vi "InitDGSystems from CnfgFile HW.vi"(8 "error in":errorcluster, 10 "Dir Calibration files":path, 11 "Config File":path) -> (0 "Errors":errorcluster[](array[cluster]), 1 "new Modules.cal?":bool, 2 "Problem Chnls out":string[](array[string]), 3 "DG Systems":refnum<class "BME_DG_System.lvclass">[](array[class]), 4 "ChnlNames":string[](array[string]), 5 "SystemNames":string[](array[string]))   [LabVIEW 2009, in "POLARIS BME DG.lvlib" / "BME_DG_System.lvclass"]
doc: "VI reads configration file and\n - reserves memory for all installed DGs\n - initializes all found systems\n - calibrates all DGs from Modules.cal\n\nOutput:\n - Problem Chnls Out : contains names of channels, they cause inconsystence by delay formulast\n - DG Systems : Array with initialized BME_DG_Systems object\n - ChnlNames : Array with all channel names in all systems\n - new Modules.cal? : is true if new Modules.cal is created. If it is the case it may by needed to correct values inside this file."
uses:
  BME_DG_System.lvclass
  POLARIS BME DG.lvlib
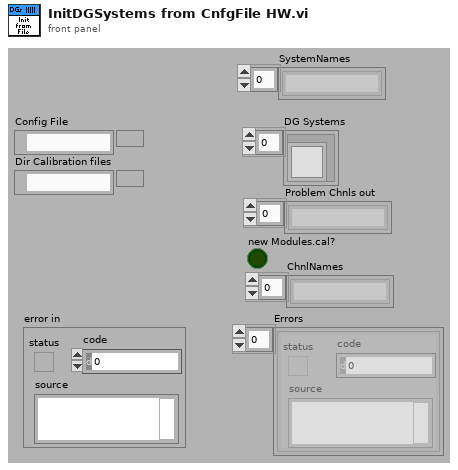
[diagram p1: front panel]
types:
  T1 = typedef "POLARIS BME DG.lvlib/BME_DG_MasterOrSlave.ctl" = enum16{"Unknown", "Master", "Slave"}
  T2 = typedef "POLARIS BME DG.lvlib/System DG Selection.ctl" = cluster{"Selected System DGs":T3[], "Name":string}
  T3 = typedef "POLARIS BME DG.lvlib/DetectDG.ctl" = cluster{"DG_Number":i32, "DG_Product":i32, "Product Name":string, "Bus_Number":i32, "Slot_Number":i32, "Master":bool}
  T4 = typedef "POLARIS BME DG.lvlib/Card Config.ctl" = cluster{"Logical Name":string, "Base Settings":T5, "SG08_Settings":T7, "Channel Names":string[], "Advanced Settings":T8}
  T5 = typedef "POLARIS BME DG.lvlib/BME_DG_TriggerSettings.ctl" = cluster{"Clock Source":T6, " clock modulo":u32, "TriggerEnabled?":bool, "trigger modulo ":i32, "InputTerminated?":bool, "Inhibit(µs)":dbl, "TriggerLevel":dbl, "PresetValue":i32, "InternalTrigger?":bool, "InternalArm?":bool, "SWTrigger?":bool, "RisingEdge?":bool, "StopOnPreset?":bool, "ResetWhenDone?":bool, "Gate Divider":i32, "PositiveGate?":bool}
  T6 = typedef "POLARIS BME DG.lvlib/ClockSource.ctl" = i32
  T7 = typedef "POLARIS BME DG.lvlib/SG08_Settings.ctl" = cluster{"Gate Terminate":bool, "Gate Level":dbl, "Gate Delay (µs)":dbl, "StepBackTime (µs)":dbl, "Burst Counter":u32, "Trigger Divider":u32, "Trigger Multiplier":u32}
  T8 = typedef "POLARIS BME DG.lvlib/BME_DG_V2TriggerSettings.ctl" = cluster{"Trigger on MS Bus":T9, "Force Trigger (µs)":dbl, "Gate Type":bool, "Synchronize Gate":bool}
  T9 = typedef "POLARIS BME DG.lvlib/MSBusSignals.ctl" = u32
  T10 = typedef "POLARIS BME DG.lvlib/Chnl Settings Complete.ctl" = cluster{"Channel Name":string, "ChnParameter":T11, "DelayFormula":string, "OutputModulo":i32, "Go and Done Signal":T12, "G08_Chnl_Settings":T14}
  T11 = typedef "POLARIS BME DG.lvlib/ChnlSettings.ctl" = cluster{" Delay (µs)":dbl, "On?":bool, "PositiveVoltage?":bool, "50OhmTerminated? ":bool, "25OhmOutput?":bool}
  T12 = typedef "POLARIS BME DG.lvlib/Go_Done_Chnl_Settings.ctl" = cluster{"Go Signal":T13, "Done Signal":u32}
  T13 = typedef "POLARIS BME DG.lvlib/GoSignalBits.ctl" = u32
  T14 = typedef "POLARIS BME DG.lvlib/SG08_Chnl_Settings.ctl" = cluster{"Pulse Width (µs)":dbl, "Output Offset":u32, "Disconnect (E,F)":bool, "Onto MsBus (E,F)":bool, "Input Positive (E,F)":bool}
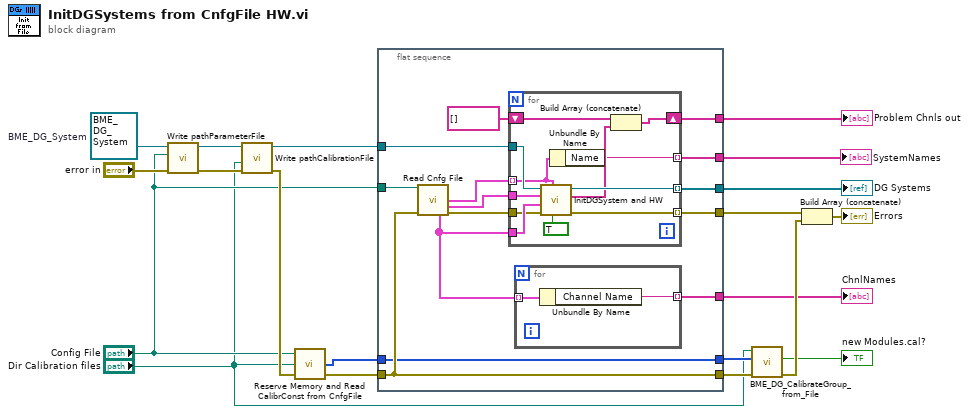
[diagram p0: block diagram]
diagram:
  w18 = refnum<class "BME_DG_System.lvclass"> refnum  # BME_DG_System
  n1 = call-dynamic "Write pathParameterFile.vi"("error in (no error)"="error in", "pathParameterFile"="Config File", "BME_DG_System in"=w18) -> ("error out"=w9:errorcluster, "BME_DG_System out"=w10:refnum<class "BME_DG_System.lvclass">)  [unwired: 7 in]
  n2 = call-dynamic "Write pathCalibrationFile.vi"("error in (no error)"=w9, "pathModulesCal"="Dir Calibration files", "BME_DG_System in"=w10) -> ("error out"=w8:errorcluster, "BME_DG_System out"=w11:refnum<class "BME_DG_System.lvclass">)  [unwired: 7 in]
  n3 = call "Reserve Memory and Read CalibrConst from CnfgFile.vi"("error in"=w8, "pathCalibrConsts"="Dir Calibration files", "pathConfigFile"="Config File") -> ("error out"=w17:errorcluster, "Master or Slave?"=w15:T1[])  [unwired: 1 in]
  n4 = flat-sequence {
    tunnel: [w31] -> w20
    tunnel: [w30] -> w19
    tunnel: w11 -> [w29]
    tunnel: w17 -> [w27]
    tunnel: "Config File" -> [w28]
    tunnel: [w27] -> w16
    tunnel: [w26] -> w14
    tunnel: w15 -> [w26]
    tunnel: [w25] -> w4
    tunnel: [w22] -> w3
    tunnel: [w21] -> w1
    frame #0 {
      n5 = call "Read Cnfg File.vi"("Config File"=w28, "error in (no error)"=w27) -> ("DGSystems"=w34:T2[], "Cards"=w32:T4[], "Chnls"=w23:T10[], "error out"=w33:errorcluster)  [unwired: 8 in, 2 out]
      n6 = for {
        tunnel: w34 -> [w38] mode=indexing
        tunnel: w33 -> [w46]
        tunnel: w32 -> [w48]
        tunnel: w23 -> [w47]
        tunnel: [w45] -> w30 mode=indexing
        tunnel: [w44] -> w31 mode=indexing
        tunnel: w29 -> [w43]
        shift-right: [w40] -> w25
        shift-left: string[] [] ("Problem Chnls out") -> [w42]
        tunnel: [w37] -> w21 mode=indexing
        n7 = call "InitDGSystem and HW.vi"("InitHW(false)"=TRUE, "System"=w38, "error in"=w46, "Chnls"=w47, "Cards"=w48, "BME_DG_System in"=w43) -> ("error out"=w45:errorcluster, "Problem Chnls out"=w41:string[], "BME_DG_System in"=w44:refnum<class "BME_DG_System.lvclass">)  [unwired: 3 in]
        n8 = Unbundle By Name(w38) -> ("Name"=w37:string)
        n9 = Build Array (concatenate)(w42, w41) -> (w40:string[])
      }
      n10 = for {
        tunnel: w23 -> [w36] mode=indexing
        tunnel: [w35] -> w22 mode=indexing
        n11 = Unbundle By Name(w36) -> ("Channel Name"=w35:string)
      }
    }
  }
  n12 = call "BME_DG_CalibrateGroup_from_File.vi"("error in (no error)"=w16, "p_MasterOrSlave"=w14, "Path"="Dir Calibration files") -> ("error out"=w12:errorcluster, "Created new"=→"new Modules.cal?":bool)  [unwired: 7 in]
  n13 = Build Array (concatenate)(w19, w12) -> (→"Errors":errorcluster[])
  "DG Systems" <- w20
  "Problem Chnls out" <- w4
  "ChnlNames" <- w3
  "SystemNames" <- w1
